vi "LMS on New GIC E.vi"(8 "Iteration num":dbl, 11 "GIC Input":T1={"     Use ?\nOff       On"=[FALSE, TRUE, FALSE, TRUE], "Mode:"=FALSE, "Extra Port"="", "Hokuyo Port"="COM7", "Tx Prop  Port"="COM6", "Compass Port"="", "GPS Port"="", "Num of WPs"=0, "WP Lats and Longs"={"WP Lats"=[], "WP Longs"=[]}, "Obst Lats and Longs"={"Obst Lats"=[], "Obst Longs"=[]}, "Parameters"=[], "GPS Data"=[], "Compass"=0.0, "LMS Vector"=[], "Vision Vector"=[], "Direction Cmd"=0.0, "Speed Cmd"=0.0, "WP Vector"=[], "WP Number"=0, "Extra"=0, "SW Map"=[], "Path Cluster"={"Path x node"=[], "Path y node"=[]}, "Sim Course"=[]} {"Obst Lats and Longs"."Obst Longs" format="%#_8g"; "Obst Lats and Longs"."Obst Lats" format="%#_8g"}) -> (3 "GIC Output":T1={"     Use ?\nOff       On"=[FALSE, TRUE, FALSE, TRUE], "Mode:"=FALSE, "Extra Port"="", "Hokuyo Port"="COM7", "Tx Prop  Port"="COM6", "Compass Port"="", "GPS Port"="", "Num of WPs"=0, "WP Lats and Longs"={"WP Lats"=[], "WP Longs"=[]}, "Obst Lats and Longs"={"Obst Lats"=[], "Obst Longs"=[]}, "Parameters"=[], "GPS Data"=[], "Compass"=0.0, "LMS Vector"=[], "Vision Vector"=[], "Direction Cmd"=0.0, "Speed Cmd"=0.0, "WP Vector"=[], "WP Number"=0, "Extra"=0, "SW Map"=[], "Path Cluster"={"Path x node"=[], "Path y node"=[]}, "Sim Course"=[]} {"Obst Lats and Longs"."Obst Longs" format="%#_8g"; "Obst Lats and Longs"."Obst Lats" format="%#_8g"})   [LabVIEW 2014]
uses:
  Hokuyo URG Series.lvlib
panel:
  in  "End Point":dbl=135.0
  in  "Start Point":dbl=-135.0
  in  "Cluster Count":dbl=1.0
  in  "Encoding Width":u16(ring)=3 items=["2 Byte"=2, "3 Byte"=3]
  in  "Scan Interval":dbl
  in  "Number of Scans":dbl
  out "swmap":dbl[][](array[numeric])
  out "lms vector":dbl[](array[numeric])
  # "LMS on New GIC E"
  # "Input:"
  # "Output:"
  # "Iteration input:"
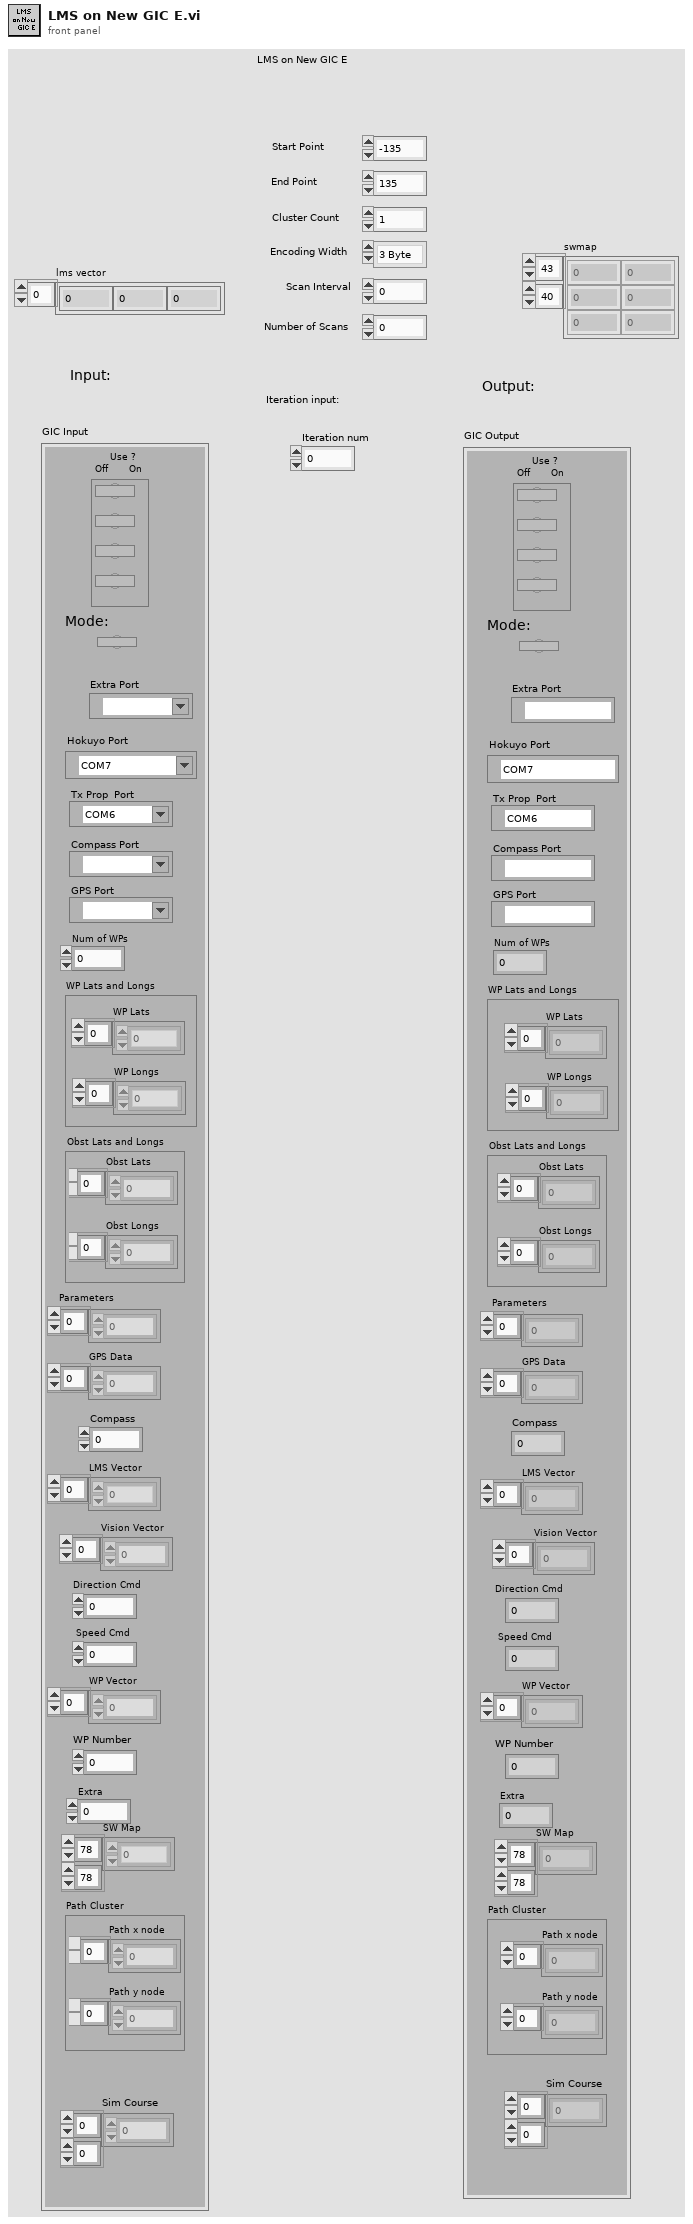
[diagram p1: front panel]
types:
  T1 = cluster{"     Use ?\nOff       On":bool[], "Mode:":bool, "Extra Port":refnum<visa-resource-name>, "Hokuyo Port":refnum<visa-resource-name>, "Tx Prop  Port":refnum<visa-resource-name>, "Compass Port":refnum<visa-resource-name>, "GPS Port":refnum<visa-resource-name>, "Num of WPs":i16, "WP Lats and Longs":cluster{"WP Lats":dbl[], "WP Longs":dbl[]}, "Obst Lats and Longs":cluster{"Obst Lats":dbl[], "Obst Longs":dbl[]}, "Parameters":dbl[], "GPS Data":dbl[], "Compass":dbl, "LMS Vector":dbl[], "Vision Vector":dbl[], "Direction Cmd":dbl, "Speed Cmd":dbl, "WP Vector":dbl[], "WP Number":i32, "Extra":i16, "SW Map":i32[][], "Path Cluster":cluster{"Path x node":dbl[], "Path y node":dbl[]}, "Sim Course":i8[][]}
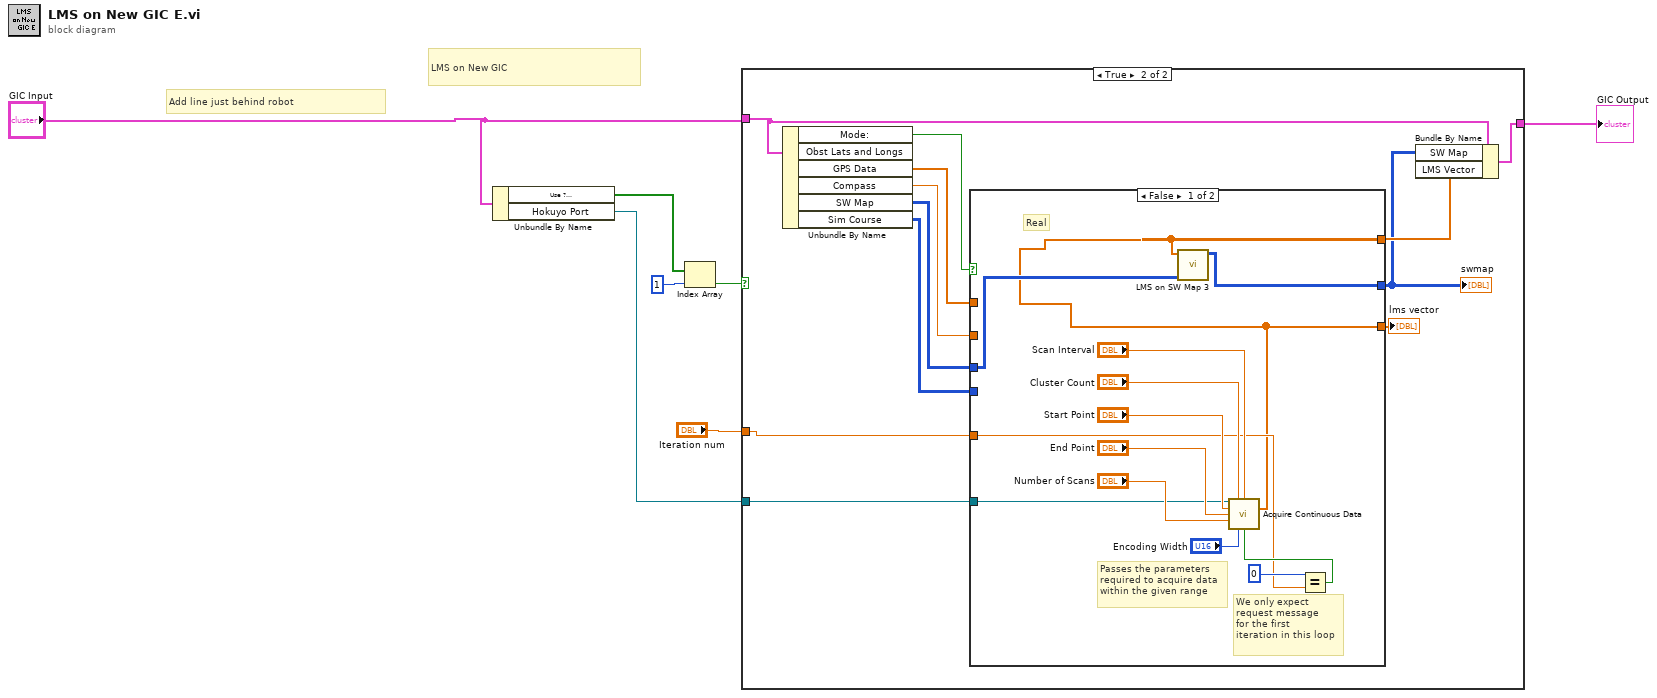
[diagram p0: block diagram]
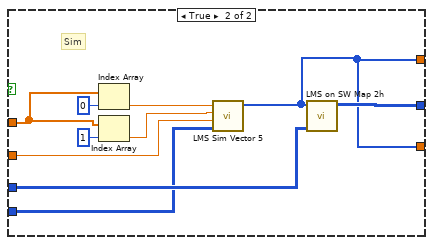
[diagram p3: hidden frame]
diagram:
  # "LMS on New GIC"
  # "Add line just behind robot"
  n1 = Unbundle By Name("GIC Input") -> ("Use ?\nOff       On"=w7:bool[], "Hokuyo Port"=w2:refnum<visa-resource-name>)
  n2 = Index Array(array=w7, index=1) -> (element=w3:bool)
  n3 = case shown="True" w3 {
    tunnel: "GIC Input" -> [w8 w16]
    tunnel: [w8 w13] -> w5
    tunnel: w2 -> [_ w12]
    tunnel: "Iteration num" -> [_ w10]
    frame False {
    }
    frame True {
      n4 = Unbundle By Name(w16) -> ("Mode:"=w20:bool, "GPS Data"=w19:dbl[], "Compass"=w18:dbl, "SW Map"=w15:i32[][], "Sim Course"=w9:i8[][])  [unwired: 1 out]
      n5 = case shown="False" w20 {
        tunnel: w19 -> [_ w38]
        tunnel: w18 -> [_ w35]
        tunnel: w15 -> [w23 w43]
        tunnel: [w22 w42] -> w11
        tunnel: [w21 w41] -> w17
        tunnel: [w21 w41] -> w14
        tunnel: w12 -> [w27 _]
        tunnel: w10 -> [w24 _]
        tunnel: w9 -> [_ w34]
        frame False {
          # "We only expect\nrequest message\nfor the first\niteration in this loop"
          # "Passes the parameters\nrequired to acquire data\nwithin the given range"
          # "Real"
          n6 = Equal?(x=0, y=w24) -> (x = y?=w25:bool)
          n7 = call "Acquire Continuous Data.vi"("VISA resource name"=w27, "Cluster Count (1)"="Cluster Count", "Scan Interval (1)"="Scan Interval", "Start Point (-120°)"="Start Point", "End Point (120°)"="End Point", "Number of Scans (0)"="Number of Scans", "Data Encoding Width (3 Byte)"="Encoding Width", "Enable Request Message (F:Disable)"=w25) -> ("Magnitude"=w21:dbl[])  [unwired: 2 in, 5 out]
          n8 = call "LMS on SW Map 3.vi"("SW Map In"=w23, "LMS Vector"=w21) -> ("SW Map Out"=w22:i32[][])  [unwired: 9 in]
        }
        frame True {
          # "Sim"
          n9 = Index Array(array=w38, index=0) -> (element=w40:dbl)
          n10 = Index Array(array=w38, index=1) -> (element=w36:dbl)
          n11 = call "LMS Sim Vector 5.vi"("Sim Course"=w34, "Robot Heading"=w35, "Robot Long"=w36, "Robot Lat"=w40) -> ("dist"=w41:i32[])  [unwired: 7 in]
          n12 = call "LMS on SW Map 2h.vi"("SW Map In"=w43, "LMS Vector"=w41) -> ("SW Map Out"=w42:i32[][])  [unwired: 9 in]
        }
      }
      "lms vector" <- w14
      "swmap" <- w11
      n13 = Bundle By Name(cluster=w16, "SW Map"=w11, "LMS Vector"=w17) -> (w13:T1)
    }
  }
  "GIC Output" <- w5
